vi "KE622x -- 2182 -A Set Digital Filter Type.vi"(0 "622x Resource In":refnum<visa-resource-name>, 1 "Check For SCPI Errors? (T)":bool=TRUE, 7 "Filter Type":enum16{"Movin", "Repeat"}(ring), 11 "error in (no error)":errorcluster) -> (4 "622x Resource Out (dupl)":refnum<visa-resource-name>, 15 "error out":errorcluster)   [LabVIEW 2013, in "Keithly user program.lvlib"]
uses:
  Keithly user program.lvlib
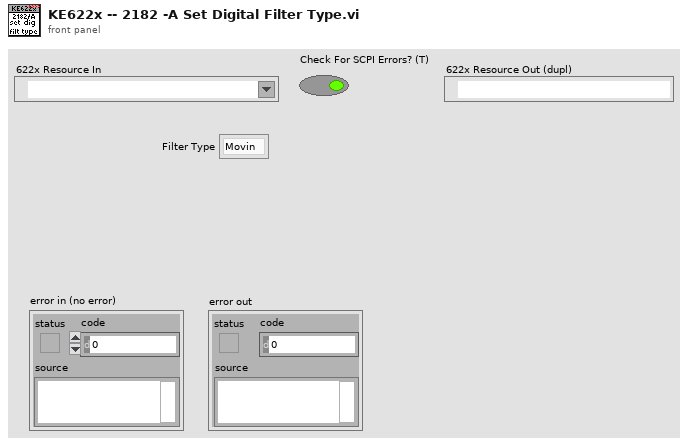
[diagram p1: front panel]
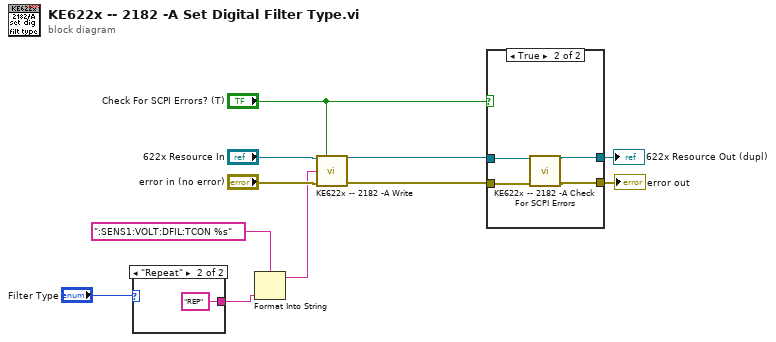
[diagram p0: block diagram]
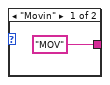
[diagram p2: hidden frame]
diagram:
  n1 = case shown="\"Repeat\"" "Filter Type" {
    tunnel: ["MOV" "REP"] -> w8
    frame "Movin" {
    }
    frame "Repeat" {
    }
  }
  n2 = Format Into String(format string=":SENS1:VOLT:DFIL:TCON %s", w8) -> (resulting string=w2:string)  [unwired: 2 in, 1 out]
  n3 = call "KE622x -- 2182 -A Write.vi"("Resource In"="622x Resource In", "Check For SCPI Errors? (T)"="Check For SCPI Errors? (T)", "2182-A Write String"=w2, "error in (no error)"="error in (no error)") -> ("Resource Out (dupl)"=w6:refnum<visa-resource-name>, "error out"=w3:errorcluster)  [unwired: 10 in]
  n4 = case shown="True" "Check For SCPI Errors? (T)" {
    tunnel: w6 -> [w15 w19]
    tunnel: w3 -> [w14 w17]
    tunnel: [w15 w18] -> w11
    tunnel: [w14 w16] -> w10
    frame False {
    }
    frame True {
      n5 = call "KE622x -- 2182 -A Check For SCPI Errors.vi"("VISA Resource In"=w19, "error in (no error)"=w17) -> ("VISA Resource Out (dupl)"=w18:refnum<visa-resource-name>, "error out"=w16:errorcluster)  [unwired: 10 in, 2 out]
    }
  }
  "622x Resource Out (dupl)" <- w11
  "error out" <- w10
